vi "Refresh Refresh Token.vi"() -> ()   [LabVIEW 2019]
uses:
  20c1f13c-04b1-4444-99e9-c77c844bb109.vi
  6ef2c51b-76d8-436a-9c2f-9e77d7ac0b1f.vi
  <vilib>/JDP Science/JSONtext/Find Item.vi
  <vilib>/JDP Science/JSONtext/String Subset.vi
  globals.vi
  <vilib>/httpClient/POSTBuffer.vi
  <vilib>/JDP Science/JSONtext/Parsing/Parse Full Path or Item Name.vi
  <vilib>/JDP Science/JSONtext/Next JSON Value.vi
  <vilib>/JDP Science/JSONtext/support/Error Cluster From Code.vi
  <vilib>/JDP Science/JSONtext/Offset/Find Item Locations by Path.vi
  <vilib>/JDP Science/JSONtext/JSON text to Variant.vi
  <vilib>/JDP Science/JSONtext/LVClass Serializer/JSONtext LVClass Serializer.lvclass
  Useful OAuth VIs.lvlib
  <vilib>/httpClient/LabVIEWHTTPClient.lvlib
  <vilib>/wsapi/NI_WebServices.lvlib
panel:
  in  "Number of days to refresh":u32=13
  out "error out":errorcluster
  in  "Redirect URI":string="http://localhost:8001/OAuth/Redirect"
  in  "Client Secret":string="Tx~D4BO32ip_x~_salD8.nHFyC7XIXCKuI"
  in  "Scopes (separated by single space)":string="offline_access Notes.ReadWrite"
  in  "Client ID":string="6224e1bc-8db0-4ef6-9504-7e49f93fdd78"
  in  "Tenant Type":string="organizations"
  in  "Error In (No Error)":errorcluster
  out "access token":string caption="<JSON>Item"
  out "Request body":string
  out "Request URI":string
  out "headers":string
  out "token response (JSON)":string
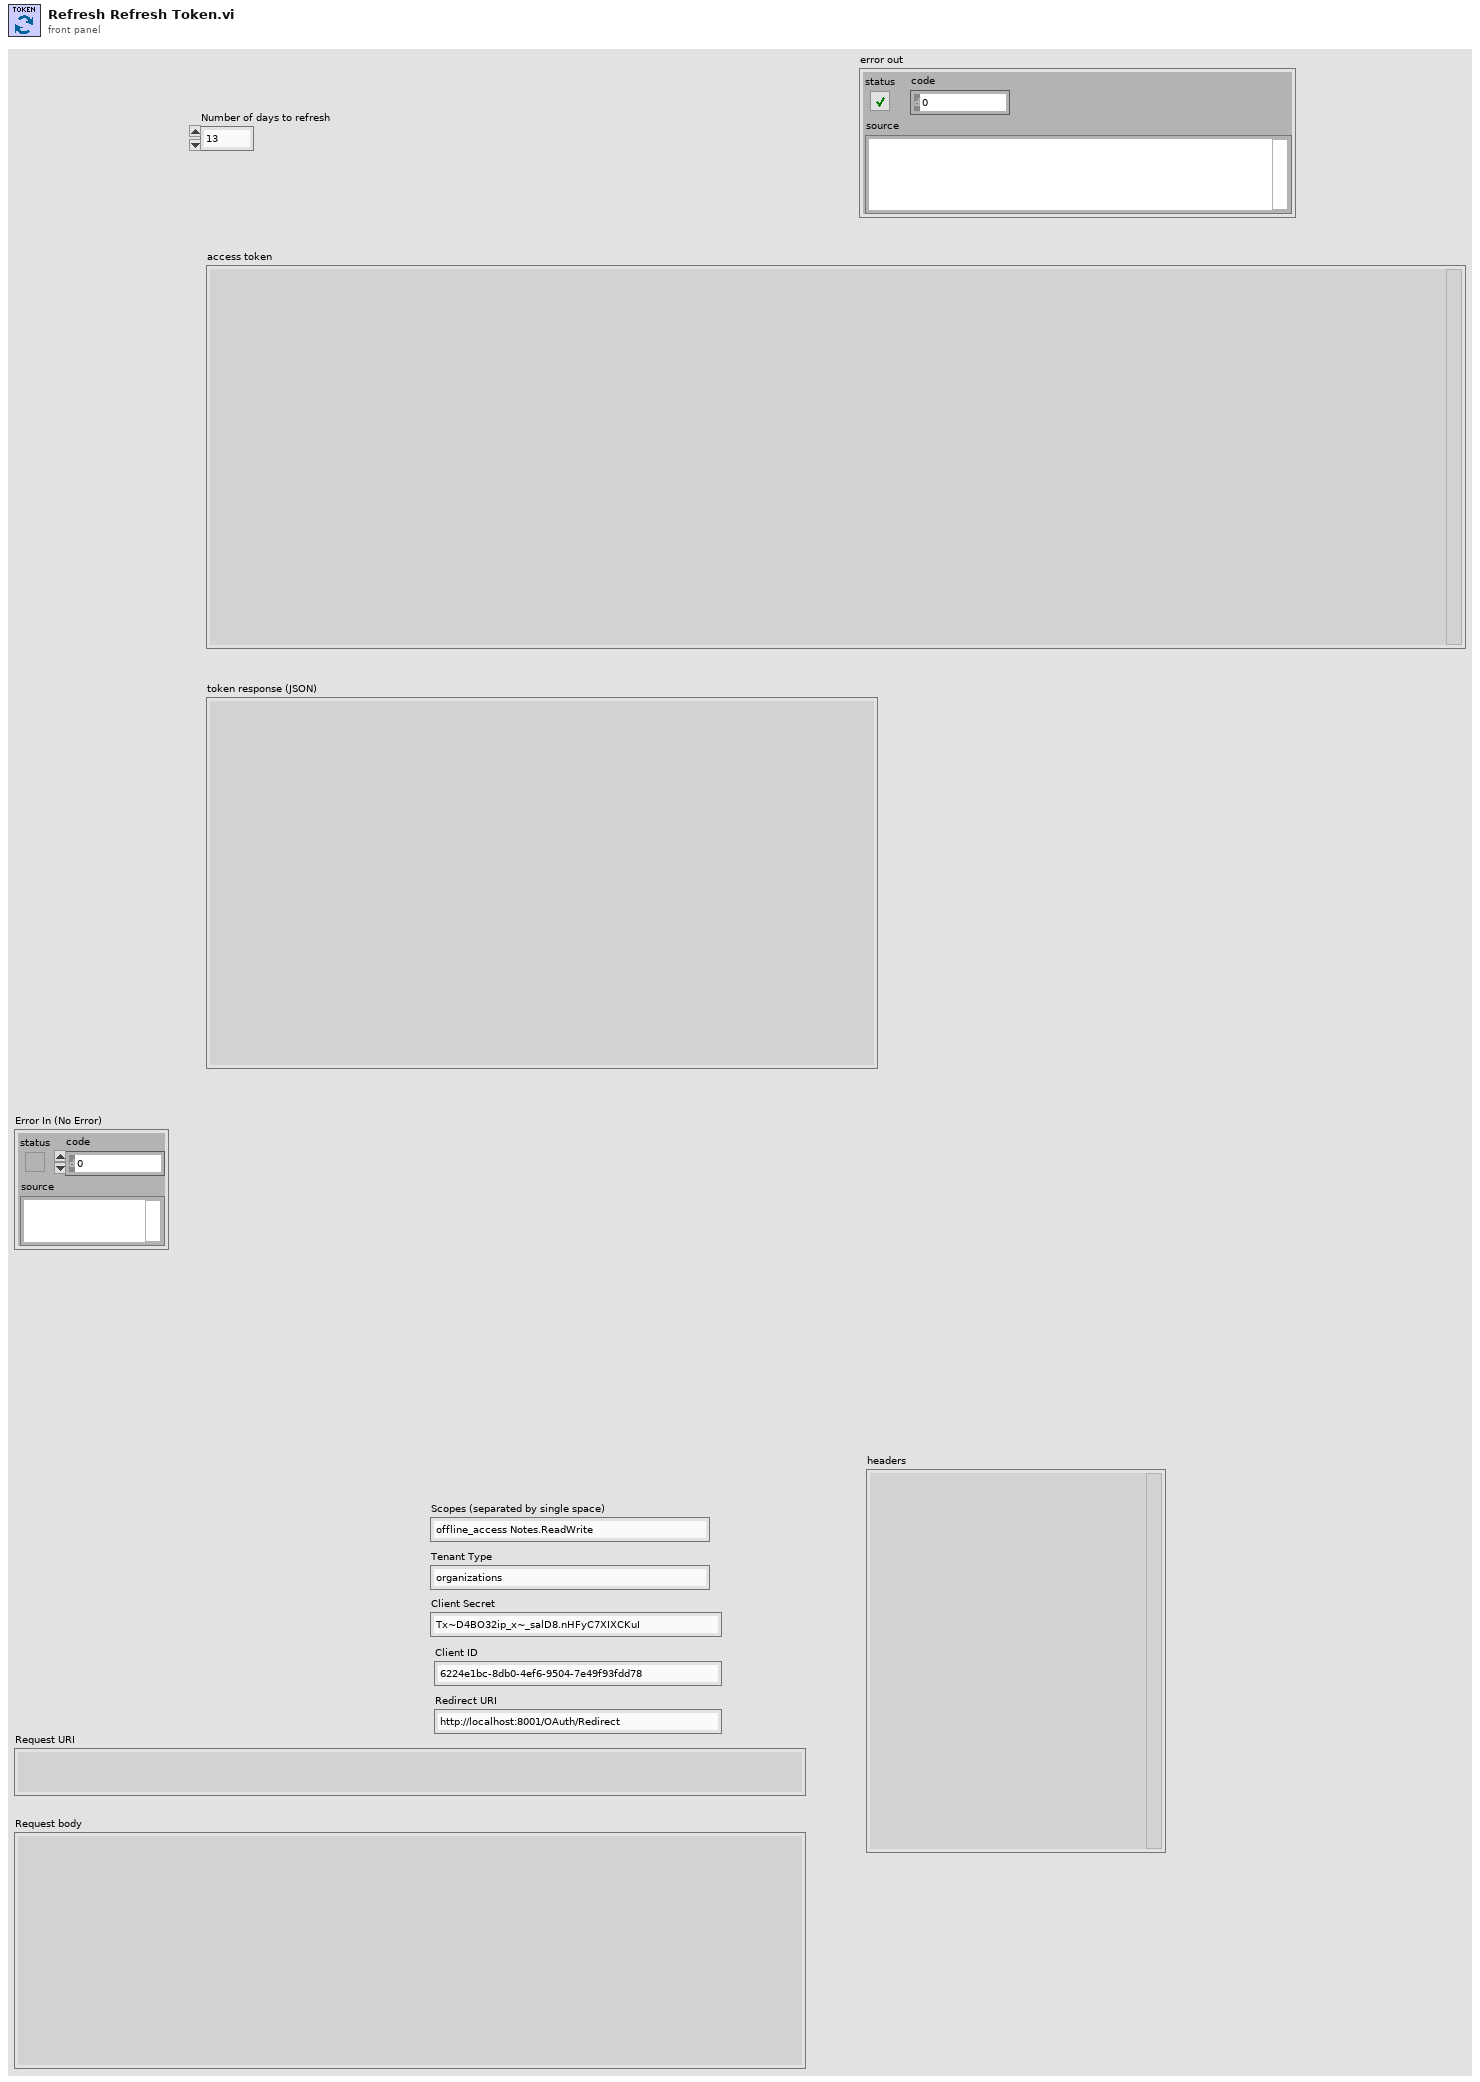
[diagram p1: front panel]
types:
  T1 = typedef "LabVIEWHTTPClient.lvlib/ClientHandle.ctl" = refnum<k1>
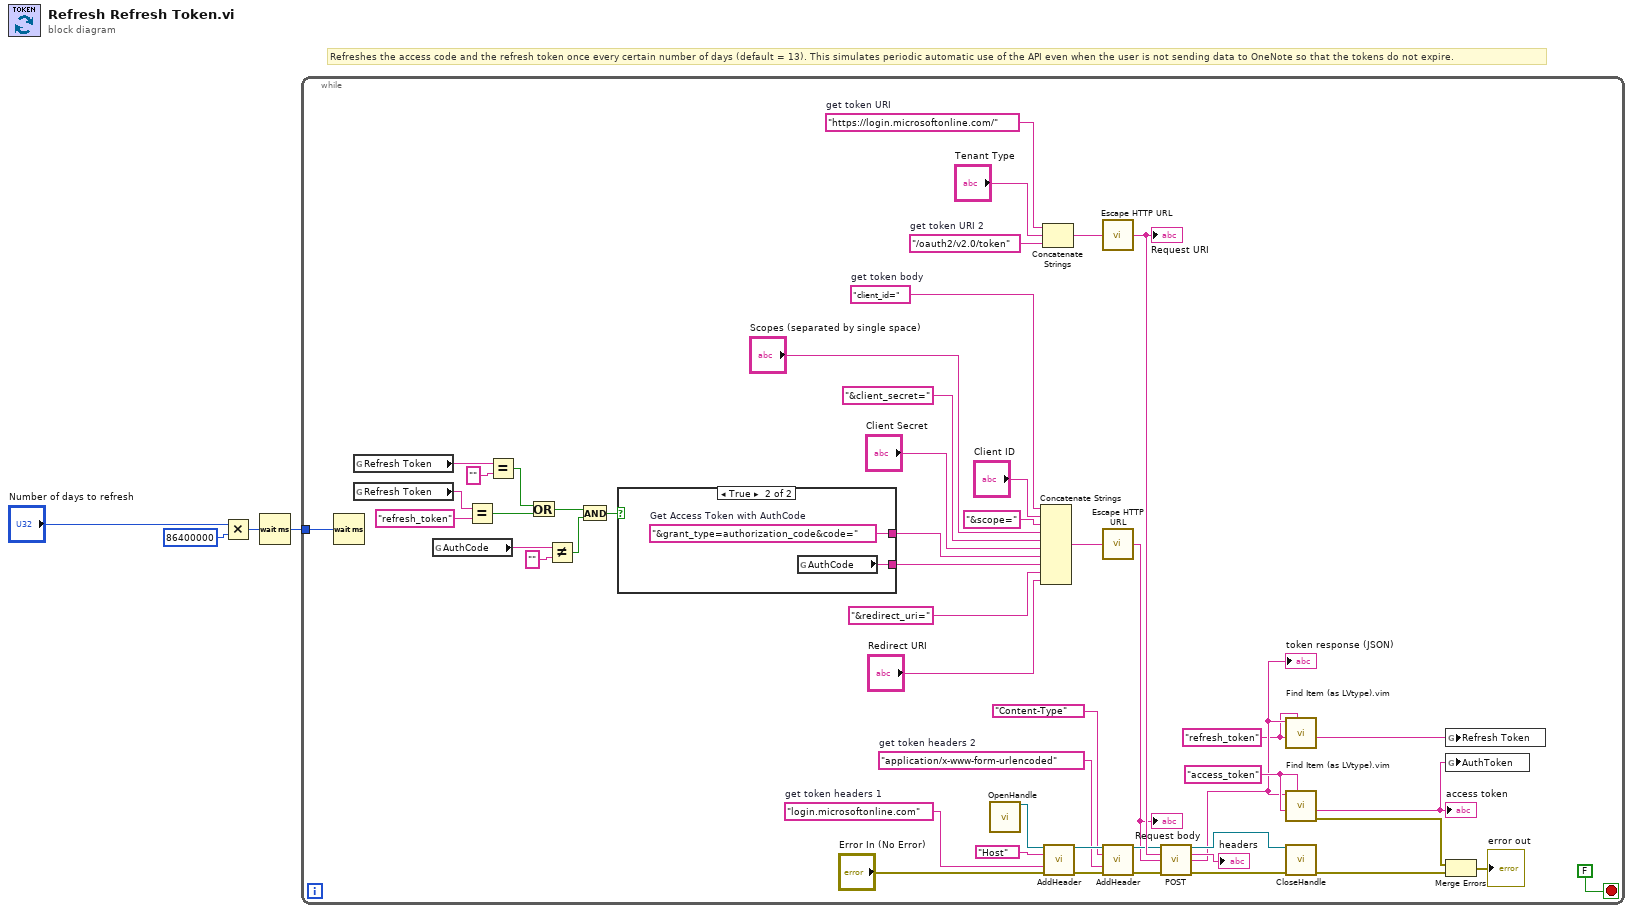
[diagram p0: block diagram]
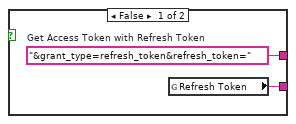
[diagram p2: hidden frame]
diagram:
  # "Refreshes the access code and the refresh token once every certain number of days (default = 13). This simulates periodic automatic use of the API even when the user is not sending data to OneNote so that the tokens do not expire."
  n1 = Multiply(x="Number of days to refresh", y=u32 86400000) -> (x*y=w2:u32)
  n2 = Wait (ms)(milliseconds to wait=w2) -> (millisecond timer value=w1:u32)
  n3 = while {
    tunnel: w1 -> [w5]
    stop <- FALSE stop-if-true
    w19 = "refresh_token" ("$Path or Item Name")
    w40 = "access_token" ("key")
    w44 = "application/x-www-form-urlencoded"  # get token headers 2
    w46 = "login.microsoftonline.com"  # get token headers 1
    w53 = "/oauth2/v2.0/token"  # get token URI 2
    w51 = "https://login.microsoftonline.com/"  # get token URI
    w42 = "client_id="  # get token body
    n4 = Wait (ms)(milliseconds to wait=w5) -> ()  [unwired: 1 out]
    n5 = global read "globals.vi" "Refresh Token"() -> (w11:string)
    n6 = global read "globals.vi" "Refresh Token"() -> (w17:string)
    n7 = global read "globals.vi" "AuthCode"() -> (w15:string)
    n8 = Equal?(x=w17, y="refresh_token") -> (x = y?=w8:bool)
    n9 = Equal?(x=w11, y="") -> (x = y?=w9:bool)
    n10 = Or(x=w9, y=w8) -> (x .or. y?=w7:bool)
    n11 = Not Equal?(x=w15, y="") -> (x != y?=w13:bool)
    n12 = And(x=w7, y=w13) -> (x .and. y?=w12:bool)
    n13 = case shown="True" w12 {
      tunnel: [w57 w59] -> w38
      tunnel: [w56 w58] -> w22
      frame False {
        w57 = "&grant_type=refresh_token&refresh_token="  # Get Access Token with Refresh Token
        n14 = global read "globals.vi" "Refresh Token"() -> (w56:string)
      }
      frame True {
        w59 = "&grant_type=authorization_code&code="  # Get Access Token with AuthCode
        n15 = global read "globals.vi" "AuthCode"() -> (w58:string)
      }
    }
    n16 = call <vilib>:"OpenHandle.vi"() -> ("client handle out"=w31:T1)  [unwired: 14 in, 1 out]
    n17 = Concatenate Strings(w42, "Client ID", "&scope=" ("string"), "Scopes (separated by single space)", "&client_secret=" ("string"), "Client Secret", w38, w22, "&redirect_uri=" ("string"), "Redirect URI") -> (w37:string)
    n18 = Concatenate Strings(w51, "Tenant Type", w53) -> (w52:string)
    n19 = call <vilib>:"AddHeader.vi"("client handle"=w31, "header"="Host", "value"=w46, "error in (no error)"="Error In (No Error)") -> ("client handle out"=w55:T1, "error out"=w54:errorcluster)  [unwired: 10 in]
    n20 = call <vilib>:"Escape HTTP URL.vi"("unescaped string in"=w52) -> ("escaped string out"=w50:string)
    "Request URI" <- w50
    n21 = call <vilib>:"Escape HTTP URL.vi"("unescaped string in"=w37) -> ("escaped string out"=w36:string)
    "Request body" <- w36
    n22 = call <vilib>:"AddHeader.vi"("client handle"=w55, "header"="Content-Type", "value"=w44, "error in (no error)"=w54) -> ("client handle out"=w43:T1, "error out"=w48:errorcluster)  [unwired: 10 in]
    n23 = call-poly <vilib>:"POST.vi"("client handle"=w43, "url"=w50, "buffer"=w36, "error in (no error)"=w48) -> ("client handle out"=w30:T1, "headers"=→"headers":string, "body"=w20:string, "error out"=w28:errorcluster)  [unwired: 8 in]
    "token response (JSON)" <- w20
    n24 = call "Find Item (as LVtype).vim"("$Path or Item Name"=w19, "Data Type and Default Value"=w19, "JSON"=w20) -> ("Data"=w18:string)  [unwired: 5 in, 3 out]
    n25 = call "Find Item (as LVtype).vim"("$Path or Item Name"=w40, "Data Type and Default Value"=w40, "JSON"=w20) -> ("error out"=w39:errorcluster, "Data"=w21:string)  [unwired: 5 in, 2 out]
    "access token" <- w21
    n26 = call <vilib>:"CloseHandle.vi"("client handle"=w30, "error in (no error)"=w28) -> ("error out"=w29:errorcluster)  [unwired: 13 in]
    n27 = global write "globals.vi" "Refresh Token"(w18) -> ()
    n28 = global write "globals.vi" "AuthToken"(w21) -> ()
    n29 = Merge Errors(w39, w29) -> (→"error out":errorcluster)
  }
